vi "Test Data.vi"(8 "error in (no error)":errorcluster, 11 "Instrument.Lockin in":refnum<class "Instrument.Lockin.lvclass">) -> (0 "error out":errorcluster, 3 "Instrument.Lockin out":refnum<class "Instrument.Lockin.lvclass">)   [LabVIEW 2019]
uses:
  src/Instrument.Lockin/Instrument.Lockin.lvclass
  <vilib>/addons/_JKI Toolkits/Caraya/classes/Assert/Assert Not Error.vi
  <vilib>/addons/_JKI Toolkits/Caraya/classes/Assert/Assert False.vi
  <vilib>/addons/_JKI Toolkits/Caraya/classes/Test/Test.lvclass
  <vilib>/addons/_JKI Toolkits/Caraya/classes/Assert/Assert.lvclass
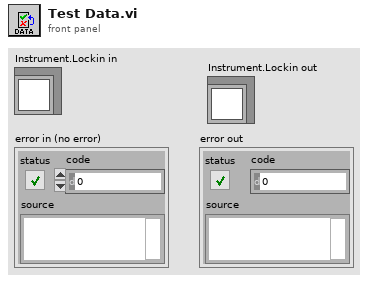
[diagram p1: front panel]
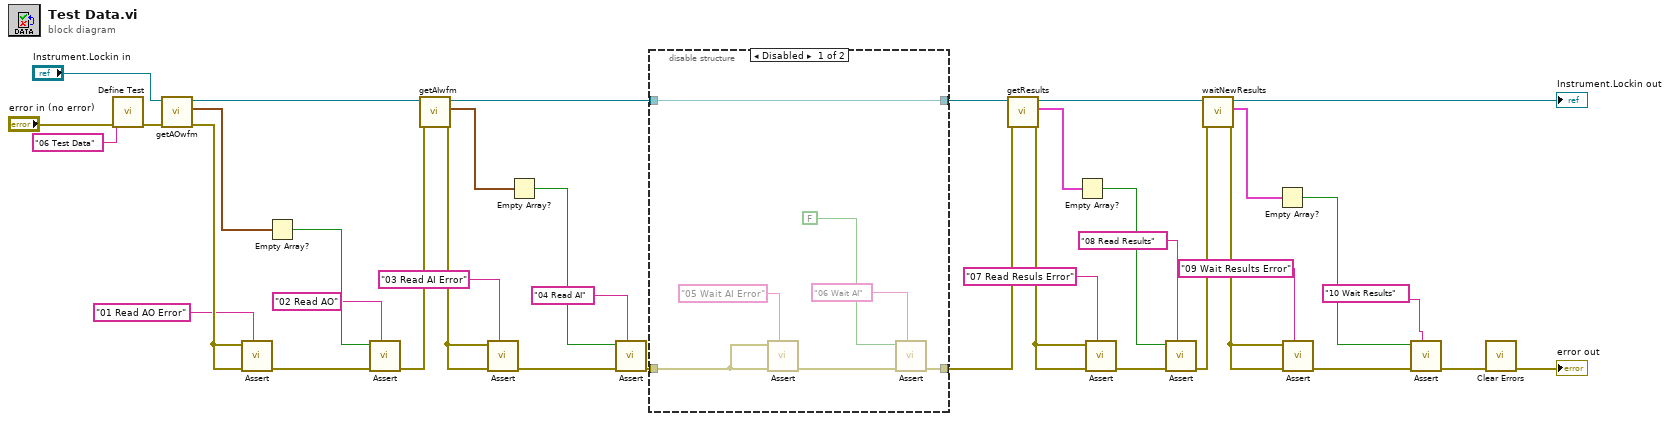
[diagram p0: block diagram]
diagram:
  n1 = call <vilib>:"Define Test.vi"("error in (no error)"="error in (no error)", "Label (VI Title)"="06 Test Data") -> ("error out"=w36:errorcluster)  [unwired: 8 in, 1 out]
  n2 = call-dynamic "getAOwfm.vi"("error in (no error)"=w36, "Instrument.Lockin in"="Instrument.Lockin in") -> ("error out"=w12:errorcluster, "AO Waveforrm"=w35:waveform(dbl)[], "Instrument.Lockin out"=w8:refnum<class "Instrument.Lockin.lvclass">)  [unwired: 7 in]
  n3 = call-poly <vilib>:"Assert.vi"("Label"="01 Read AO Error", "error in (no error)"=w12, "Not Error?"=w12) -> ("error out"=w29:errorcluster)  [unwired: 7 in, 1 out]
  n4 = Empty Array?(array=w35) -> (empty?=w28:bool)
  n5 = call-poly <vilib>:"Assert.vi"("Label"="02 Read AO", "error in (no error)"=w29, "False?"=w28) -> ("error out"=w27:errorcluster)  [unwired: 7 in, 1 out]
  n6 = call-dynamic "getAIwfm.vi"("error in (no error)"=w27, "Instrument.Lockin in"=w8) -> ("error out"=w26:errorcluster, "AI Waveform"=w34:waveform(dbl)[], "Instrument.Lockin out"=w7:refnum<class "Instrument.Lockin.lvclass">)  [unwired: 7 in]
  n7 = call-poly <vilib>:"Assert.vi"("Label"="03 Read AI Error", "error in (no error)"=w26, "Not Error?"=w26) -> ("error out"=w25:errorcluster)  [unwired: 7 in, 1 out]
  n8 = Empty Array?(array=w34) -> (empty?=w23:bool)
  n9 = call-poly <vilib>:"Assert.vi"("Label"="04 Read AI", "error in (no error)"=w25, "False?"=w23) -> ("error out"=w14:errorcluster)  [unwired: 7 in, 1 out]
  n10 = disable-structure shown="Disabled" {
    disable-tunnel: w14 -> [w42 w47]
    disable-tunnel: [w44 w47] -> w13
    disable-tunnel: w7 -> [w41 w48]
    disable-tunnel: [w41 w48] -> w6
    frame Disabled {
      n11 = call-poly <vilib>:"Assert.vi"("Label"="05 Wait AI Error", "error in (no error)"=w42, "Not Error?"=w42) -> ("error out"=w46:errorcluster)  [unwired: 7 in, 1 out]
      n12 = call-poly <vilib>:"Assert.vi"("Label"="06 Wait AI", "error in (no error)"=w46, "False?"=FALSE) -> ("error out"=w44:errorcluster)  [unwired: 7 in, 1 out]
    }
    frame Enabled {
    }
  }
  n13 = call-dynamic "getResults.vi"("error in (no error)"=w13, "Instrument.Lockin in"=w6) -> ("error out"=w21:errorcluster, "Results (Dictionary)"=w33:cluster{"key":string, "value":dbl}[], "Instrument.Lockin out"=w2:refnum<class "Instrument.Lockin.lvclass">)  [unwired: 6 in, 1 out]
  n14 = Empty Array?(array=w33) -> (empty?=w20:bool)
  n15 = call-poly <vilib>:"Assert.vi"("Label"="07 Read Resuls Error", "error in (no error)"=w21, "Not Error?"=w21) -> ("error out"=w22:errorcluster)  [unwired: 7 in, 1 out]
  n16 = call-poly <vilib>:"Assert.vi"("Label"="08 Read Results", "error in (no error)"=w22, "False?"=w20) -> ("error out"=w15:errorcluster)  [unwired: 7 in, 1 out]
  n17 = call-dynamic "waitNewResults.vi"("error in (no error)"=w15, "Instrument.Lockin in"=w2) -> ("error out"=w19:errorcluster, "Results (Dictionary)"=w32:cluster{"key":string, "value":dbl}[], "Instrument.Lockin out"=→"Instrument.Lockin out":refnum<class "Instrument.Lockin.lvclass">)  [unwired: 7 in]
  n18 = Empty Array?(array=w32) -> (empty?=w17:bool)
  n19 = call-poly <vilib>:"Assert.vi"("Label"="09 Wait Results Error", "error in (no error)"=w19, "Not Error?"=w19) -> ("error out"=w18:errorcluster)  [unwired: 7 in, 1 out]
  n20 = call-poly <vilib>:"Assert.vi"("Label"="10 Wait Results", "error in (no error)"=w18, "False?"=w17) -> ("error out"=w16:errorcluster)  [unwired: 7 in, 1 out]
  n21 = call <vilib>:"Clear Errors.vi"("error in (no error)"=w16) -> ("error out"=→"error out":errorcluster)  [unwired: 5 in, 1 out]
